vi "init.vi"   [LabVIEW 2017]
doc: "refer：消息队列实例\nsize：默认-1，无限大\nname：队列名称，可以是字符或者非空字符数组，数组元素不得重复，生成字符数组大小的消息队列数组。"
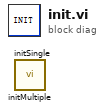
[diagram p0: block diagram]
diagram:
  n1 = call "initMultiple.vi"() -> ()  [unwired: 10 in, 2 out]
  n2 = call "initSingle.vi"() -> ()  [unwired: 10 in, 2 out]
